vi "DBC Get Msg Name.vi"(9 "pMsgName":string, 10 "index":i32, 11 "DBCHandle":u64) -> (1 "pMsgName out":string, 3 "function return":i32)   [LabVIEW 2010, in "dbc_parser.lvlib"]
doc: "int WINAPI DBC_GetMsgName(long long DBCHandle, int index, char* pMsgName);"
uses:
  dbc_parser.lvlib
  USB2XXX/trunk/USB2XXX/USB2XXX/vs2019/Release/USB2XXX.dll
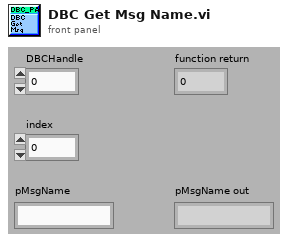
[diagram p1: front panel]
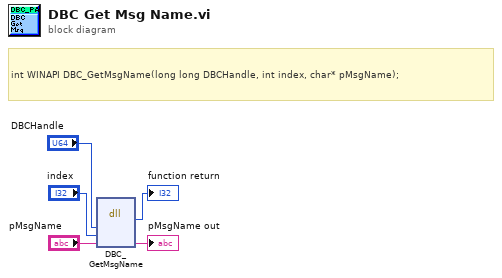
[diagram p0: block diagram]
diagram:
  # "int WINAPI DBC_GetMsgName(long long DBCHandle, int index, char* pMsgName);"
  n1 = dll-call lib="E:/Projects/USB2XXX/trunk/USB2XXX/USB2XXX/vs2019/Release/USB2XXX.*" fn="DBC_GetMsgName"("DBCHandle"="DBCHandle", "index"="index", "pMsgName"="pMsgName") -> (→"function return":i32, "pMsgName"=→"pMsgName out":string)  [unwired: 5 in, 2 out]
